vi "settings_from_XML_singleVI.vi"(0 "XML in":string, 1 "vi reference":refnum<vi>) -> (3 "VI":string, 4 "Version":string, 5 "vi reference out":refnum<vi>)   [LabVIEW 2015]
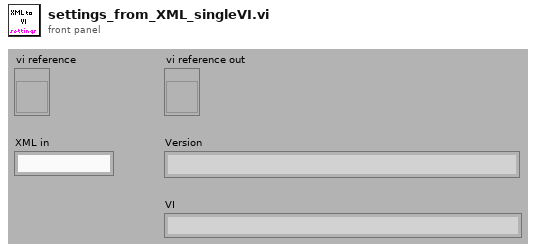
[diagram p1: front panel]
types:
  T1 = cluster{"Name":string, "Version":string, "Controls":cluster{"Name":string, "Data":string}[]}
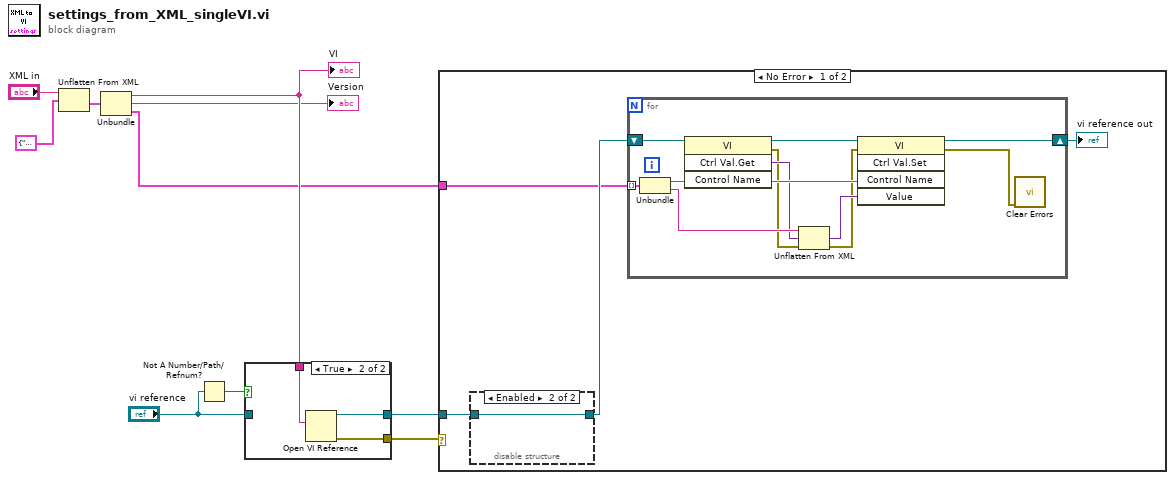
[diagram p0: block diagram]
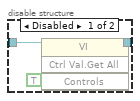
[diagram p2: hidden frame]
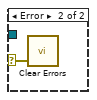
[diagram p3: hidden frame]
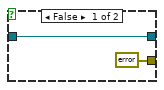
[diagram p4: hidden frame]
diagram:
  n1 = Unflatten From XML(xml string="XML in", type=T1 {"Name"="", "Version"="", "Controls"=[]} ("cluster")) -> (value=w4:T1)  [unwired: 1 in, 1 out]
  n2 = Unbundle(w4) -> ("Name"=w3:string, "Version"=→"Version":string, "Controls"=w1:cluster{"Name":string, "Data":string}[])
  "VI" <- w3
  n3 = Not A Number/Path/Refnum?(number/path/refnum="vi reference") -> (NaN/Path/Refnum?=w10:bool)
  n4 = case shown="True" w10 {
    tunnel: "vi reference" -> [w11 _]
    tunnel: [w11 w15] -> w8
    tunnel: w3 -> [_ w14]
    tunnel: [errorcluster {"status"=FALSE, "code"=0, "source"=""} ("error out") w13] -> w7
    frame False {
    }
    frame True {
      n5 = Open VI Reference(vi path=w14) -> (vi reference=w15:refnum<vi>, error out=w13:errorcluster)  [unwired: 5 in]
    }
  }
  n6 = case shown="No Error" w7 {
    selector: w7 -> [_ w35]
    tunnel: w1 -> [w16 _]
    tunnel: w8 -> [w17 _]
    frame No Error {
      n7 = disable-structure shown="Enabled" {
        disable-tunnel: [w22 w23] -> w19
        disable-tunnel: w17 -> [w20 w23]
        frame Disabled {
          n8 = invoke class="VI" method="Ctrl Val.Get All"(reference=w20, "Controls"=TRUE) -> (reference out=w22:refnum<vi>)  [unwired: 2 in, 3 out]
        }
        frame Enabled {
        }
      }
      n9 = for {
        tunnel: w16 -> [w31] mode=indexing
        shift-right: [w34] -> w18
        shift-left: w19 -> [w28]
        n10 = Unbundle(w31) -> ("Name"=w29:string, "Data"=w32:string)
        n11 = invoke class="VI" method="Ctrl Val.Get"(reference=w28, "Control Name"=w29) -> (reference out=w27:refnum<vi>, error out=w25:errorcluster, "Get Control Value Variant"=w26:variant)  [unwired: 2 in, 1 out]
        n12 = Unflatten From XML(xml string=w32, type=w26, error in (no error)=w25) -> (value=w30:variant, error out=w24:errorcluster)
        n13 = invoke class="VI" method="Ctrl Val.Set"(reference=w27, error in=w24, "Control Name"=w29, "Value"=w30) -> (reference out=w34:refnum<vi>, error out=w33:errorcluster)  [unwired: 1 in, 3 out]
        n14 = call <vilib>:"Clear Errors.vi"("error in (no error)"=w33) -> ()  [unwired: 5 in, 2 out]
      }
      "vi reference out" <- w18
    }
    frame Error {
      n15 = call <vilib>:"Clear Errors.vi"("error in (no error)"=w35) -> ()  [unwired: 5 in, 2 out]
    }
  }
